vi "generateEvent.vi"(8 "error in":errorcluster, 11 "command":enum16{"ini", "get", "close"}(ring)=enum."get") -> (0 "error out":errorcluster, 3 "tcp data event":T1)   [LabVIEW 2011]
uses:
  tcp_new_data_event.ctl
  tcp new data cluster.ctl
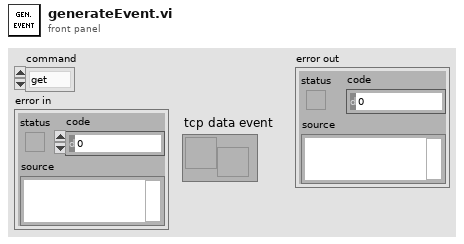
[diagram p1: front panel]
types:
  T1 = typedef "tcp_new_data_event.ctl" = refnum<user-event>
  T2 = typedef "tcp new data cluster.ctl" = cluster{"EventEnum":enum16{"new data", "connection status update"}, "Device name":string}
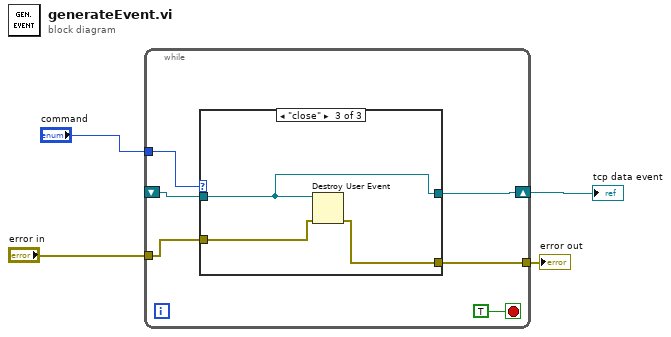
[diagram p0: block diagram]
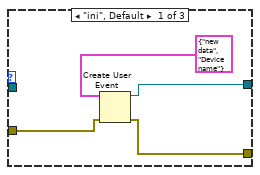
[diagram p2: hidden frame]
diagram:
  n1 = while {
    tunnel: "command" -> [w10]
    shift-right: [w9] -> w3
    shift-left: _ -> [w8]
    tunnel: [w7] -> w1
    tunnel: "error in" -> [w6]
    stop <- TRUE stop-if-true
    n2 = case shown="\"close\"" w10 {
      tunnel: [w13 w16 w19] -> w9
      tunnel: w8 -> [_ w16 w19]
      tunnel: w6 -> [w12 w15 w18]
      tunnel: [w11 w15 w17] -> w7
      frame "ini", Default {
        n3 = Create User Event(user event datatype=T2 {"EventEnum"=enum."new data", "Device name"="Device name"} ("New Event"), error in=w12) -> (user event=w13:refnum<user-event>, error out=w11:errorcluster)
      }
      frame "get" {
      }
      frame "close" {
        n4 = Destroy User Event(user event=w19, error in=w18) -> (error out=w17:errorcluster)
      }
    }
  }
  "tcp data event" <- w3
  "error out" <- w1
